vi "Command.vi"(8 "error in (no error)":errorcluster, 10 "Http Chan Cmd":T1, 11 "HTTP Command Bridge in":refnum<class "HTTP Command Bridge.lvclass">) -> (0 "error out":errorcluster, 3 "HTTP Command Bridge out":refnum<class "HTTP Command Bridge.lvclass">)   [LabVIEW 2023, in "Volatus.lvlib" / "HTTP Command Bridge.lvclass"]
uses:
  HTTP Command Bridge.lvclass
  Http Chan Cmd.ctl
  Http Cmd Type.ctl
  HTTP Command Bridge.lvclass/HTTP Command Bridge.ctl
  messages/CmdDigital/Data.ctl
  MessageQ/MessageQ.lvclass/MessageQ.ctl
  messages/CmdDigitalMultiple/Class/Msg.lvclass/Msg.ctl
  Module/Module.lvclass/Module.ctl
  VolatusAPI/VolatusAPI.lvclass/VolatusAPI.ctl
  messages/CmdAnalog/Data.ctl
  messages/CmdAnalogMultiple/Class/Msg.lvclass/Msg.ctl
  messages/CmdDigitalMultiple/Class/Msg.lvclass
  messages/CmdAnalogMultiple/Class/Msg.lvclass
  lv-vecto/Vecto/TCPMessageService/Send Message.vi
  lv-protoc/LV-Proto/Message/Message.lvclass
  Module/Module.lvclass
  messages/CmdDigital/CmdDigital.lvlib
  VolatusAPI/VolatusAPI.lvclass
  MessageQ/MessageQ.lvclass
  C:/dev/volatus/mts-volatus-super/libs/lv-volatus/Volatus/Module/Module.lvclass
  C:/dev/volatus/mts-volatus-super/libs/lv-volatus/Volatus/HTTP Command Bridge/HTTP Command Bridge.lvclass
  messages/CmdAnalog/CmdAnalog.lvlib
  messages/CmdAnalogMultiple/CmdAnalogMultiple.lvlib
  messages/CmdDigitalMultiple/CmdDigitalMultiple.lvlib
  C:/dev/volatus/mts-volatus-super/libs/lv-volatus/messages/CmdDigitalMultiple/Class/Msg.lvclass
  C:/dev/volatus/mts-volatus-super/libs/lv-protoc/LV-Proto/Message/Message.lvclass
  C:/dev/volatus/mts-volatus-super/libs/lv-volatus/messages/CmdAnalogMultiple/Class/Msg.lvclass
  Volatus.lvlib
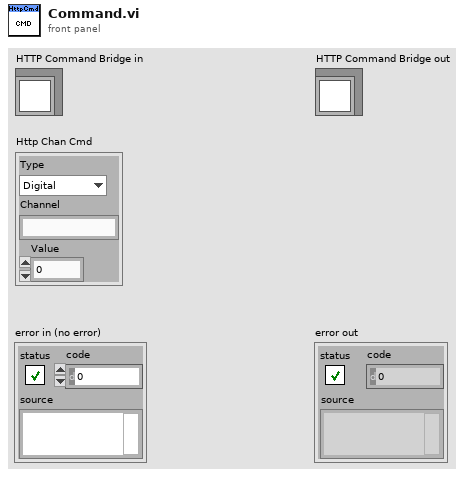
[diagram p1: front panel]
types:
  T1 = typedef "Volatus.lvlib/Http Chan Cmd.ctl" = cluster{"Type":T2, "Channel":string, "Value":dbl}
  T2 = typedef "Volatus.lvlib/Http Cmd Type.ctl" = enum16{"Digital", "Numeric"}
  T3 = typedef "Volatus.lvlib/HTTP Command Bridge.lvclass/Command Info.ctl" = cluster{"Destination":T4, "Local Q":refnum<class "MessageQ.lvclass">, "Target":string, "Task":string}
  T4 = typedef "Volatus.lvlib/HTTP Command Bridge.lvclass/Command Dest.ctl" = enum16{"Local", "Remote"}
  T5 = typedef "CmdDigital.lvlib/Data.ctl" = cluster{"channel":string, "value":bool}
  T6 = typedef "CmdAnalog.lvlib/Data.ctl" = cluster{"channel":string, "value":dbl}
  T7 = typedef "CmdDigitalMultiple.lvlib/Data.ctl" = cluster{"values":T5[]}
  T8 = typedef "CmdAnalogMultiple.lvlib/Data.ctl" = cluster{"values":T6[]}
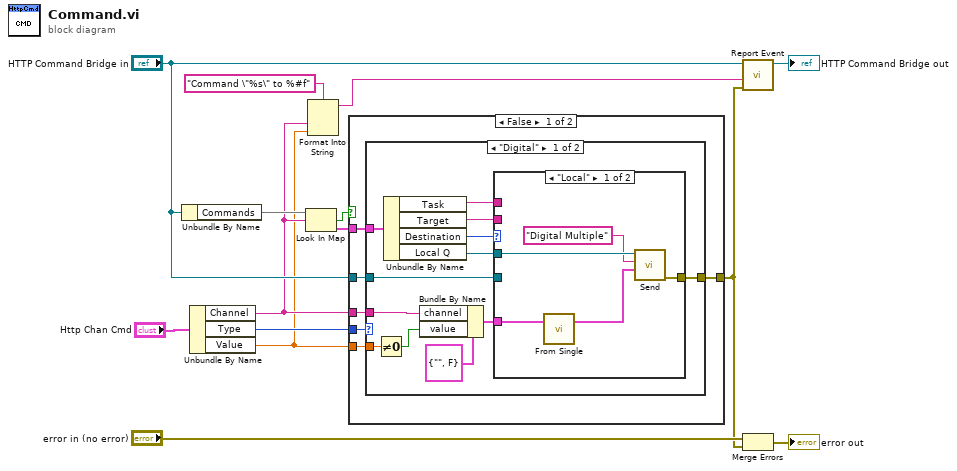
[diagram p0: block diagram]
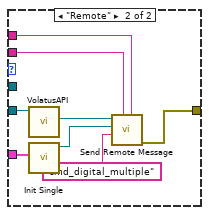
[diagram p2: hidden frame]
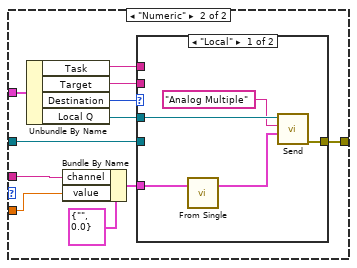
[diagram p3: hidden frame]
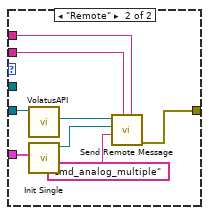
[diagram p4: hidden frame]
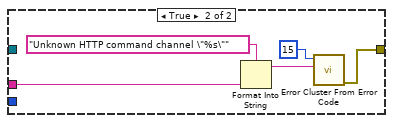
[diagram p5: hidden frame]
diagram:
  n1 = Unbundle By Name("HTTP Command Bridge in") -> ("Commands"=w13:map{string, T3})
  n2 = Unbundle By Name("Http Chan Cmd") -> ("Channel"=w4:string, "Type"=w9:T2, "Value"=w3:dbl)
  n3 = Look In Map(map=w13, key=w4) -> (key not found?=w11:bool, value=w10:T3)  [unwired: 1 in]
  n4 = Format Into String(format string="Command \"%s\" to %#f", w4, w3) -> (resulting string=w2:string)  [unwired: 2 in, 1 out]
  n5 = case shown="False" w11 {
    tunnel: w10 -> [w17 _]
    tunnel: w9 -> [w20 _]
    tunnel: w3 -> [w18 _]
    tunnel: w4 -> [w19 w70]
    tunnel: "HTTP Command Bridge in" -> [w16 _]
    tunnel: [w15 w74] -> w1
    frame False {
      n6 = case shown="\"Digital\"" w20 {
        tunnel: w19 -> [w30 w54]
        tunnel: w18 -> [w29 w53]
        tunnel: w17 -> [w27 w52]
        tunnel: w16 -> [w22 w47]
        tunnel: [w21 w46] -> w15
        frame "Digital" {
          n7 = Not Equal To 0?(x=w29) -> (x != 0?=w28:bool)
          n8 = Unbundle By Name(w27) -> ("Task"=w23:string, "Target"=w24:string, "Destination"=w26:T4, "Local Q"=w25:refnum<class "MessageQ.lvclass">)
          n9 = Bundle By Name(cluster=T5 {"channel"="", "value"=FALSE} ("Data"), "channel"=w30, "value"=w28) -> (w31:T5)
          n10 = case shown="\"Local\"" w26 {
            tunnel: w31 -> [w34 w45]
            tunnel: w25 -> [w37 _]
            tunnel: w24 -> [_ w40]
            tunnel: w23 -> [_ w39]
            tunnel: w22 -> [_ w44]
            tunnel: [w35 w38] -> w21
            frame "Local" {
              n11 = call "From Single.vi"("CmdDigital"=w34) -> ("CmdDigitalMultiple"=w33:T7)  [unwired: 6 in]
              n12 = call "Send.vi"("Data"=w33, "ID"="Digital Multiple", "MessageQ in"=w37) -> ("error out"=w35:errorcluster)  [unwired: 7 in, 1 out]
            }
            frame "Remote" {
              n13 = call "VolatusAPI.vi"("Module in"=w44) -> ("VolatusAPI"=w43:refnum<class "VolatusAPI.lvclass">)  [unwired: 9 in, 1 out]
              n14 = call "Init Single.vi"("value"=w45) -> ("Msg out"=w42:refnum<class "Msg.lvclass">)  [unwired: 10 in]
              n15 = call "Send Remote Message.vi"("Target Task (None)"=w39, "Target Name"=w40, "Message Type"="cmd_digital_multiple", "Message"=w42, "VolatusAPI in"=w43) -> ("error out"=w38:errorcluster)  [unwired: 5 in, 1 out]
            }
          }
        }
        frame "Numeric" {
          n16 = Unbundle By Name(w52) -> ("Task"=w48:string, "Target"=w49:string, "Destination"=w51:T4, "Local Q"=w50:refnum<class "MessageQ.lvclass">)
          n17 = Bundle By Name(cluster=T6 {"channel"="", "value"=0.0} ("Data"), "channel"=w54, "value"=w53) -> (w55:T6)
          n18 = case shown="\"Local\"" w51 {
            tunnel: w55 -> [w59 w69]
            tunnel: w50 -> [w61 _]
            tunnel: w49 -> [_ w64]
            tunnel: w48 -> [_ w63]
            tunnel: w47 -> [_ w68]
            tunnel: [w58 w62] -> w46
            frame "Local" {
              n19 = call "From Single.vi"("CmdAnalog"=w59) -> ("CmdAnalogMultiple"=w57:T8)  [unwired: 6 in]
              n20 = call "Send.vi"("Data"=w57, "ID"="Analog Multiple", "MessageQ in"=w61) -> ("error out"=w58:errorcluster)  [unwired: 7 in, 1 out]
            }
            frame "Remote" {
              n21 = call "VolatusAPI.vi"("Module in"=w68) -> ("VolatusAPI"=w67:refnum<class "VolatusAPI.lvclass">)  [unwired: 9 in, 1 out]
              n22 = call "Init Single.vi"("value"=w69) -> ("Msg out"=w66:refnum<class "Msg.lvclass">)  [unwired: 10 in]
              n23 = call "Send Remote Message.vi"("Target Task (None)"=w63, "Target Name"=w64, "Message Type"="cmd_analog_multiple", "Message"=w66, "VolatusAPI in"=w67) -> ("error out"=w62:errorcluster)  [unwired: 5 in, 1 out]
            }
          }
        }
      }
    }
    frame True {
      n24 = Format Into String(format string="Unknown HTTP command channel \"%s\"", w70) -> (resulting string=w72:string)  [unwired: 2 in, 1 out]
      n25 = call <vilib>:"Error Cluster From Error Code.vi"("error message (\"\")"=w72, "error code (0)"=15) -> ("error out"=w74:errorcluster)  [unwired: 7 in]
    }
  }
  n26 = call "Report Event.vi"("error in (no error)"=w1, "Message"=w2, "Module in"="HTTP Command Bridge in") -> ("Module out"=→"HTTP Command Bridge out":refnum<class "HTTP Command Bridge.lvclass">)  [unwired: 7 in, 1 out]
  n27 = Merge Errors("error in (no error)", w1) -> (→"error out":errorcluster)
